vi "kawa.vi"() -> ()   [LabVIEW 2023]
uses:
  states.ctl
  cluster.ctl
panel:
  in  "stop":bool
  out "Whipped Cream":bool
  out "Chocolate Syrup":bool
  out "Milk Foam":bool
  out "Steamed Milk":bool
  out "Espresso":bool
  in  "Cafe Mocha":bool
  in  "Caffe Latte":bool
  in  "Espresso Macchiato":bool
  in  "Espresso":bool
  # "Wybierz kawe:"
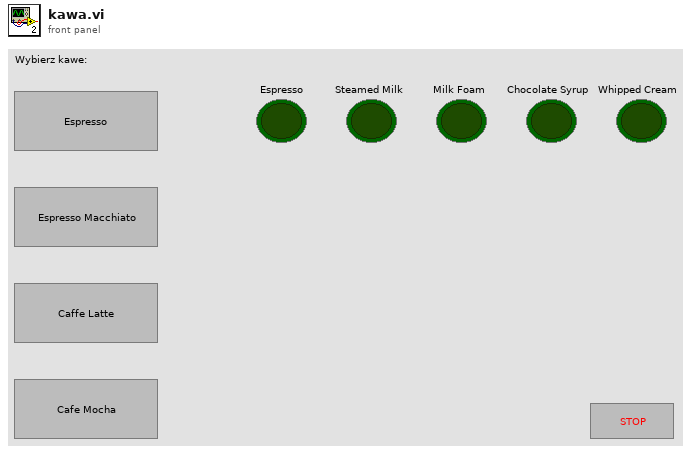
[diagram p1: front panel]
types:
  T1 = typedef "states.ctl" = enum16{"init", "idle", "coffe_init", "coffe_make", "wait", "write_to_file", "turn_off", "exit"}
  T2 = typedef "cluster.ctl" = cluster{"CurrentTime":timestamp, "CoffeType":enum16{"CafeMocha", "CaffeLatte", "EspressoMachiato", "Espresso"}, "Cluster":cluster{"Espresso":i32, "SteamedMilk":i32, "MilkFoam":i32, "ChocolateSyrup":i32, "WhippedCream":i32}, "TimeToWait":i32, "ElementPreparing":i32}
  T3 = enum16{"CafeMocha", "CaffeLatte", "EspressoMachiato", "Espresso"}
  T4 = enum16{"open", "replace", "create", "open or create", "replace or create", "replace or create with confirmation"}
  T5 = cluster{"Espresso":i32, "SteamedMilk":i32, "MilkFoam":i32, "ChocolateSyrup":i32, "WhippedCream":i32}
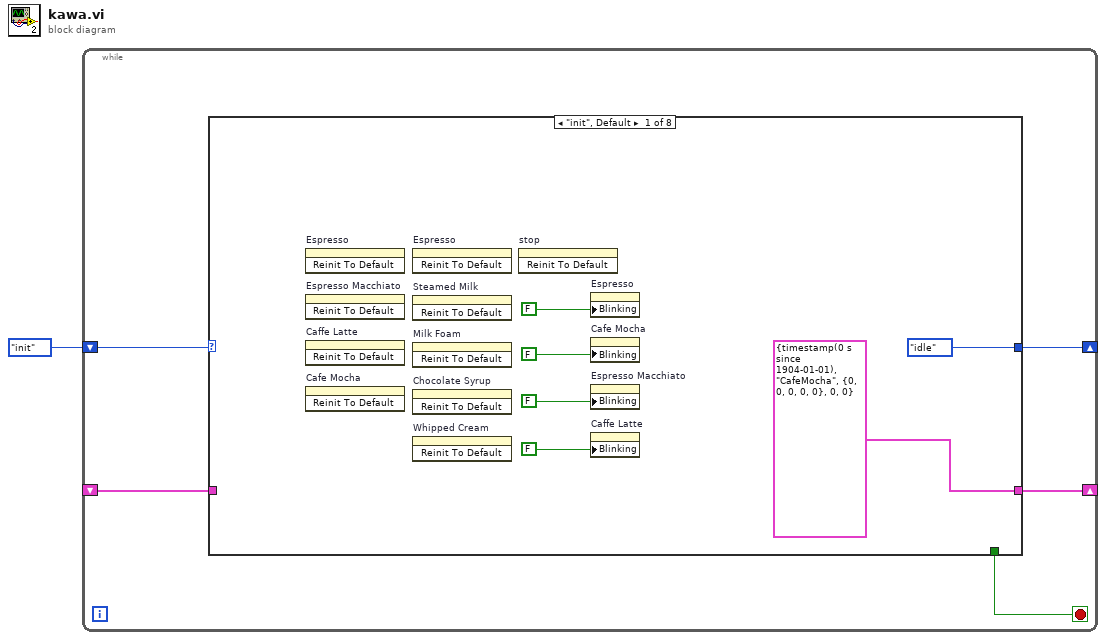
[diagram p0: block diagram]
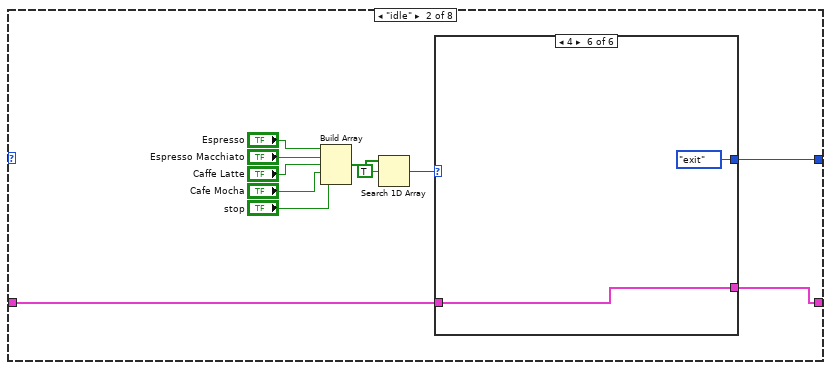
[diagram p2: hidden frame]
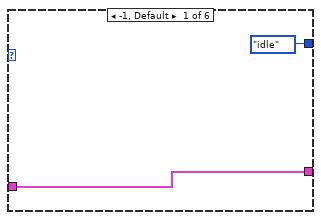
[diagram p3: hidden frame]
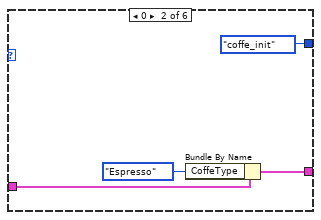
[diagram p4: hidden frame]
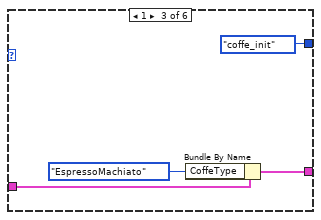
[diagram p5: hidden frame]
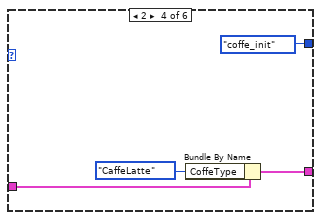
[diagram p6: hidden frame]
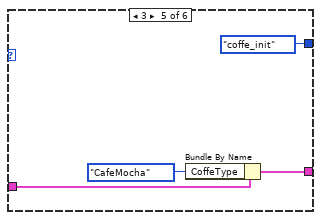
[diagram p7: hidden frame]
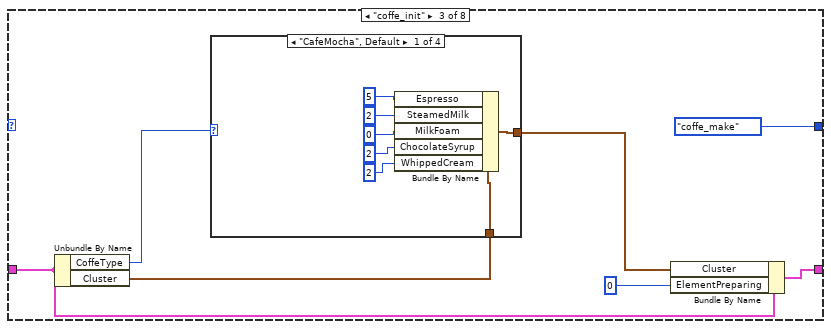
[diagram p8: hidden frame]
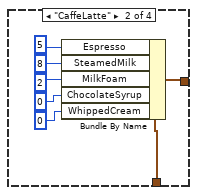
[diagram p9: hidden frame]
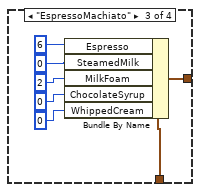
[diagram p10: hidden frame]
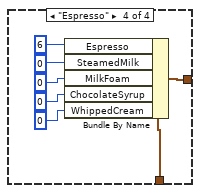
[diagram p11: hidden frame]
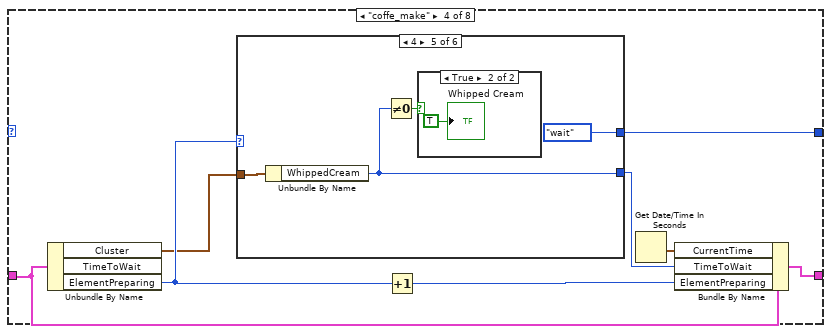
[diagram p12: hidden frame]
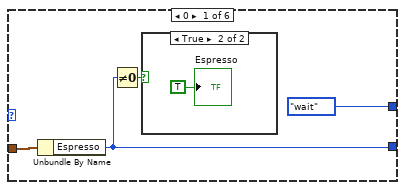
[diagram p13: hidden frame]
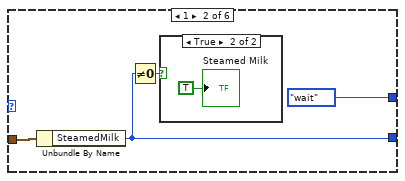
[diagram p15: hidden frame]
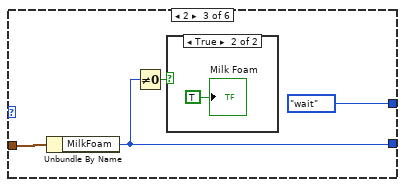
[diagram p17: hidden frame]
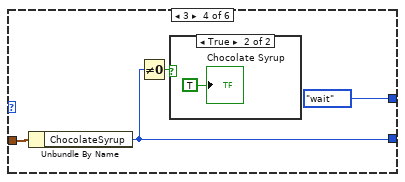
[diagram p19: hidden frame]
diagram:
  n1 = while {
    shift-right: [w5] -> _
    shift-left: states."init" ("Enum") -> [w6]
    shift-right: [w3] -> _
    shift-left: _ -> [w4]
    stop <- w2 stop-if-true
    n2 = case shown="\"init\", Default" w6 {
      tunnel: [states."idle" ("Enum") w23 states."coffe_make" ("Enum") w80 w126 states."init" ("Enum") states."coffe_make" ("Enum") states."init" ("Enum")] -> w5
      tunnel: w4 -> [_ w22 w47 w85 w125 w153 w159 w162]
      tunnel: [T2 {"CurrentTime"=timestamp(0 s since 1904-01-01), "CoffeType"=enum."CafeMocha", "Cluster"={"Espresso"=0, "SteamedMilk"=0, "MilkFoam"=0, "ChocolateSyrup"=0, "WhippedCream"=0}, "TimeToWait"=0, "ElementPreparing"=0} w21 w49 w86 w125 w153 w159 w162] -> w3
      tunnel: [_ _ _ _ _ _ _ TRUE ("stop")] -> w2
      frame "init", Default {
        n3 = invoke on="Espresso" class="Bool" method="Reinit To Default"() -> ()  [unwired: 3 in, 3 out]
        n4 = invoke on="Espresso Macchiato" class="Bool" method="Reinit To Default"() -> ()  [unwired: 3 in, 3 out]
        n5 = invoke on="Caffe Latte" class="Bool" method="Reinit To Default"() -> ()  [unwired: 3 in, 3 out]
        n6 = invoke on="Cafe Mocha" class="Bool" method="Reinit To Default"() -> ()  [unwired: 3 in, 3 out]
        n7 = invoke on="Espresso" class="Bool (strict)" method="Reinit To Default"() -> ()  [unwired: 3 in, 3 out]
        n8 = invoke on="Steamed Milk" class="Bool (strict)" method="Reinit To Default"() -> ()  [unwired: 3 in, 3 out]
        n9 = invoke on="Milk Foam" class="Bool (strict)" method="Reinit To Default"() -> ()  [unwired: 3 in, 3 out]
        n10 = invoke on="Chocolate Syrup" class="Bool (strict)" method="Reinit To Default"() -> ()  [unwired: 3 in, 3 out]
        n11 = invoke on="Whipped Cream" class="Bool (strict)" method="Reinit To Default"() -> ()  [unwired: 3 in, 3 out]
        n12 = invoke on="stop" class="Bool (strict)" method="Reinit To Default"() -> ()  [unwired: 3 in, 3 out]
        n13 = property on="Espresso" class="Bool"("Blinking"=FALSE) -> ()  [unwired: 2 in, 2 out]
        n14 = property on="Cafe Mocha" class="Bool"("Blinking"=FALSE) -> ()  [unwired: 2 in, 2 out]
        n15 = property on="Espresso Macchiato" class="Bool"("Blinking"=FALSE) -> ()  [unwired: 2 in, 2 out]
        n16 = property on="Caffe Latte" class="Bool"("Blinking"=FALSE) -> ()  [unwired: 2 in, 2 out]
      }
      frame "idle" {
        n17 = Build Array("Espresso", "Espresso Macchiato", "Caffe Latte", "Cafe Mocha", "stop") -> (w16:bool[])
        n18 = Search 1D Array(1D array=w16, element=TRUE) -> (index of element=w14:i32)  [unwired: 1 in]
        n19 = case shown="4" w14 {
          tunnel: [states."idle" ("Enum") states."coffe_init" ("Enum") states."coffe_init" ("Enum") states."coffe_init" ("Enum") states."coffe_init" ("Enum") states."exit" ("Enum")] -> w23
          tunnel: w22 -> [w24 w27 w31 w35 w39 w42]
          tunnel: [w24 w28 w32 w36 w40 w42] -> w21
          frame -1, Default {
          }
          frame 0 {
            n20 = Bundle By Name(cluster=w27, "CoffeType"=T3."Espresso" ("Enum")) -> (w28:T2)
          }
          frame 1 {
            n21 = Bundle By Name(cluster=w31, "CoffeType"=T3."EspressoMachiato" ("Enum")) -> (w32:T2)
          }
          frame 2 {
            n22 = Bundle By Name(cluster=w35, "CoffeType"=T3."CaffeLatte" ("Enum")) -> (w36:T2)
          }
          frame 3 {
            n23 = Bundle By Name(cluster=w39, "CoffeType"=T3."CafeMocha" ("Enum")) -> (w40:T2)
          }
          frame 4 {
          }
        }
      }
      frame "coffe_init" {
        n24 = Unbundle By Name(w47) -> ("CoffeType"=w48:T3, "Cluster"=w46:T5)
        n25 = case shown="\"CafeMocha\", Default" w48 {
          tunnel: [w57 w63 w71 w78] -> w44
          tunnel: w46 -> [w56 w64 w70 w77]
          frame "CafeMocha", Default {
            n26 = Bundle By Name(cluster=w56, "Espresso"=5, "SteamedMilk"=2, "MilkFoam"=0, "ChocolateSyrup"=2, "WhippedCream"=2) -> (w57:T5)
          }
          frame "CaffeLatte" {
            n27 = Bundle By Name(cluster=w64, "Espresso"=5, "SteamedMilk"=8, "MilkFoam"=2, "ChocolateSyrup"=0, "WhippedCream"=0) -> (w63:T5)
          }
          frame "EspressoMachiato" {
            n28 = Bundle By Name(cluster=w70, "Espresso"=6, "SteamedMilk"=0, "MilkFoam"=2, "ChocolateSyrup"=0, "WhippedCream"=0) -> (w71:T5)
          }
          frame "Espresso" {
            n29 = Bundle By Name(cluster=w77, "Espresso"=6, "SteamedMilk"=0, "MilkFoam"=0, "ChocolateSyrup"=0, "WhippedCream"=0) -> (w78:T5)
          }
        }
        n30 = Bundle By Name(cluster=w47, "Cluster"=w44, "ElementPreparing"=0) -> (w49:T2)
      }
      frame "coffe_make" {
        n31 = Unbundle By Name(w85) -> ("Cluster"=w82:T5, "ElementPreparing"=w84:i32)  [unwired: 1 out]
        n32 = case shown="4" w84 {
          tunnel: w82 -> [w90 w95 w100 w105 w110 _]
          tunnel: [w87 w92 w97 w102 w107 0 ("WhippedCream")] -> w81
          tunnel: [states."wait" ("Enum") states."wait" ("Enum") states."wait" ("Enum") states."wait" ("Enum") states."wait" ("Enum") states."write_to_file" ("Enum")] -> w80
          frame 0 {
            n33 = Unbundle By Name(w90) -> ("Espresso"=w87:i32)
            n34 = Not Equal To 0?(x=w87) -> (x != 0?=w88:bool)
            n35 = case shown="True" w88 {
              frame False {
              }
              frame True {
                "Espresso" <- TRUE ("Espresso")
              }
            }
          }
          frame 1 {
            n36 = Unbundle By Name(w95) -> ("SteamedMilk"=w92:i32)
            n37 = Not Equal To 0?(x=w92) -> (x != 0?=w93:bool)
            n38 = case shown="True" w93 {
              frame False {
              }
              frame True {
                "Steamed Milk" <- TRUE ("Steamed Milk")
              }
            }
          }
          frame 2 {
            n39 = Unbundle By Name(w100) -> ("MilkFoam"=w97:i32)
            n40 = Not Equal To 0?(x=w97) -> (x != 0?=w98:bool)
            n41 = case shown="True" w98 {
              frame False {
              }
              frame True {
                "Milk Foam" <- TRUE ("Milk Foam")
              }
            }
          }
          frame 3 {
            n42 = Unbundle By Name(w105) -> ("ChocolateSyrup"=w102:i32)
            n43 = Not Equal To 0?(x=w102) -> (x != 0?=w103:bool)
            n44 = case shown="True" w103 {
              frame False {
              }
              frame True {
                "Chocolate Syrup" <- TRUE ("Chocolate Syrup")
              }
            }
          }
          frame 4 {
            n45 = Unbundle By Name(w110) -> ("WhippedCream"=w107:i32)
            n46 = Not Equal To 0?(x=w107) -> (x != 0?=w108:bool)
            n47 = case shown="True" w108 {
              frame False {
              }
              frame True {
                "Whipped Cream" <- TRUE ("Whipped Cream")
              }
            }
          }
          frame 5, Default {
          }
        }
        n48 = Increment(x=w84) -> (x+1=w83:i32)
        n49 = Get Date/Time In Seconds() -> (seconds since 1Jan1904=w79:timestamp)
        n50 = Bundle By Name(cluster=w85, "CurrentTime"=w79, "TimeToWait"=w81, "ElementPreparing"=w83) -> (w86:T2)
      }
      frame "wait" {
        n51 = Unbundle By Name(w125) -> ("CurrentTime"=w123:timestamp, "CoffeType"=w116:T3, "TimeToWait"=w120:i32)  [unwired: 1 out]
        n52 = Get Date/Time In Seconds() -> (seconds since 1Jan1904=w124:timestamp)
        n53 = To Double Precision Float(number=w123) -> (double precision float=w121:dbl)
        n54 = To Double Precision Float(number=w124) -> (double precision float=w122:dbl)
        n55 = To Double Precision Float(number=w120) -> (double precision float=w118:dbl)
        n56 = Subtract(x=w122, y=w121) -> (x-y=w119:dbl)
        n57 = case shown="\"EspressoMachiato\"" w116 {
          frame "CafeMocha", Default {
            n58 = property on="Cafe Mocha" class="Bool"("Blinking"=TRUE) -> ()  [unwired: 2 in, 2 out]
          }
          frame "CaffeLatte" {
            n59 = property on="Caffe Latte" class="Bool"("Blinking"=TRUE) -> ()  [unwired: 2 in, 2 out]
          }
          frame "EspressoMachiato" {
            n60 = property on="Espresso Macchiato" class="Bool"("Blinking"=TRUE) -> ()  [unwired: 2 in, 2 out]
          }
          frame "Espresso" {
            n61 = property on="Espresso" class="Bool"("Blinking"=TRUE) -> ()  [unwired: 2 in, 2 out]
          }
        }
        n62 = Greater Or Equal?(x=w119, y=w118) -> (x >= y?=w117:bool)
        n63 = local read "stop"() -> (w114:bool)
        n64 = case shown="False" w114 {
          tunnel: [w128 states."exit" ("Enum")] -> w126
          tunnel: w117 -> [w127 _]
          frame False {
            n65 = case shown="True" w127 {
              tunnel: [states."wait" ("Enum") states."turn_off" ("Enum")] -> w128
              frame False {
              }
              frame True {
              }
            }
          }
          frame True {
          }
        }
        n66 = Wait (ms)(milliseconds to wait=u32 100) -> ()  [unwired: 1 out]
      }
      frame "write_to_file" {
        n67 = Unbundle By Name(w153) -> ("CoffeType"=w152:T3)
        n68 = case shown="\"Espresso\"" w152 {
          tunnel: ["Cafe Mocha" "Caffe Latte" "Espresso Machiato" "Espresso"] -> w143
          frame "CafeMocha", Default {
          }
          frame "CaffeLatte" {
          }
          frame "EspressoMachiato" {
          }
          frame "Espresso" {
          }
        }
        n69 = call <vilib>:"Application Directory.vi"() -> ("Application Directory"=w137:path)
        n70 = Get Date/Time String() -> (date string=w142:string, time string=w140:string)  [unwired: 3 in]
        n71 = call <vilib>:"Space Constant.vi"() -> ("String"=w141:string)
        n72 = Concatenate Strings(w143, w141, w142, w141, w140, "\r\n") -> (w145:string)
        n73 = Build Path(base path=w137, name or relative path=path "coffe.txt") -> (appended path=w138:path)
        n74 = Open/Create/Replace File(file path (use dialog)=w138, operation (0:open)=T4."open or create") -> (refnum out=w150:refnum<file>, error out=w149:errorcluster)  [unwired: 4 in, 1 out]
        n75 = Read from Text File(file (use dialog)=w150, error in=w149) -> (refnum out=w146:refnum<file>, error out=w151:errorcluster)  [unwired: 2 in, 2 out]
        n76 = Write to Text File(file (use dialog)=w146, text=w145, error in=w151) -> (refnum out=w147:refnum<file>, error out=w148:errorcluster)  [unwired: 1 in, 1 out]
        n77 = Close File(refnum=w147, error in=w148) -> ()  [unwired: 2 out]
      }
      frame "turn_off" {
        n78 = invoke on="Chocolate Syrup" class="Bool (strict)" method="Reinit To Default"() -> ()  [unwired: 3 in, 3 out]
        n79 = invoke on="Espresso" class="Bool (strict)" method="Reinit To Default"() -> ()  [unwired: 3 in, 3 out]
        n80 = invoke on="Milk Foam" class="Bool (strict)" method="Reinit To Default"() -> ()  [unwired: 3 in, 3 out]
        n81 = invoke on="Steamed Milk" class="Bool (strict)" method="Reinit To Default"() -> ()  [unwired: 3 in, 3 out]
        n82 = invoke on="Whipped Cream" class="Bool (strict)" method="Reinit To Default"() -> ()  [unwired: 3 in, 3 out]
      }
      frame "exit" {
      }
    }
  }
